vi "Send Quad Arrays to Sqlite.vi"(5 "Savepoint name":string="MySavepoint", 6 "Path to local database file *.db":path=path "C:/sqlite/sensor_data.db", 7 "TIME 1D Array REAL":dbl[](array[numeric]), 8 "error in (no error)":errorcluster, 9 "DENS 1D Array REAL":dbl[](array[numeric]), 10 "TEMP 1D Array REAL":dbl[](array[numeric]), 11 "PRESSURE 1D Array REAL":dbl[](array[numeric])) -> (0 "error out":errorcluster, 3 "Rows (Samples) Detected in input array":i32=1000)   [LabVIEW 2023]
uses:
  <vilib>/drjdpowell/SQLite Library/SQL Statement/SQL Statement.lvclass/SQL Statement.ctl
  <vilib>/drjdpowell/SQLite Library/SQL Connection/Open (path).vi
  <vilib>/drjdpowell/SQLite Library/SQL Statement/Bind Real.vi
  <vilib>/drjdpowell/SQLite Library/SQL Connection/Open (string).vi
  <vilib>/drjdpowell/SQLite Library/SQL Statement/Step.vi
  <vilib>/AdvancedString/Path To Command Line String.vi
  <vilib>/drjdpowell/SQLite Library/SQL Connection/Execute SQL (No results).vi
  <vilib>/drjdpowell/SQLite Library/SQL Statement/Error Message.vi
  <vilib>/drjdpowell/SQLite Library/SQL Connection/Connection.lvclass
  <vilib>/drjdpowell/SQLite Library/SQLite.lvlib
  <vilib>/drjdpowell/SQLite Library/Transaction Helpers/Transaction.lvlib
  <vilib>/drjdpowell/SQLite Library/SQL Statement/SQL Statement.lvclass
panel:
  in  "SQLite Command":string="CREATE TABLE IF NOT EXISTS pipe_data(\nID INTEGER PRIMARY KEY AUTOINCREMENT,\nUNIX_TIME REAL NOT NULL, \nPRESSURE REAL NOT NULL,\nTEMPERATURE REAL NOT NULL,\nDENSITY REAL NOT NULL\n);"
  # "Create a pipe_data table in sensor_data.db\nNO Indexing in this evolution.\nAdd 4 columns for data of type REAL"
  # "DATA SOURCE SELECT"
  # "THIS VI SENDS (4) 1D parameter arrays TO SQLite DATABASE TABLE pipe_data\nIt creates the table if it doesnt exist, and populates the column data with pipe parameters.\n\nAll parameter columns are forced to a NOT NULL state, any attempt at writing NULL or NaN will throw an error.\n\nNOT SURE WHAT YOU WANT TO DO ON INDEXING IN THE DB....WE CAN USE NO INDEX, INDEX ON unix_time, OR ADD A KEY FIELD. lETS DISCUSS ???????????\n\nThe first time through, the table pipe_data is created and populated with 25 samples of rando parameters.The UNIX_TIME var is not random, and should align with real times.\nThe Authority for timestamping should rest on the DAQ process to maintain accuracy, and is included in the incoming 2d array. This vi simply pushes that array time to SQLite.\nIf you run this vi again after the table has been created, the data is appended to the database in increments of 25 rows.\n\n\n\nRegarding the 14 day flush....Do you want the stale data removed from the incoming 2D array, the database, or both ?\nThroughput ?"
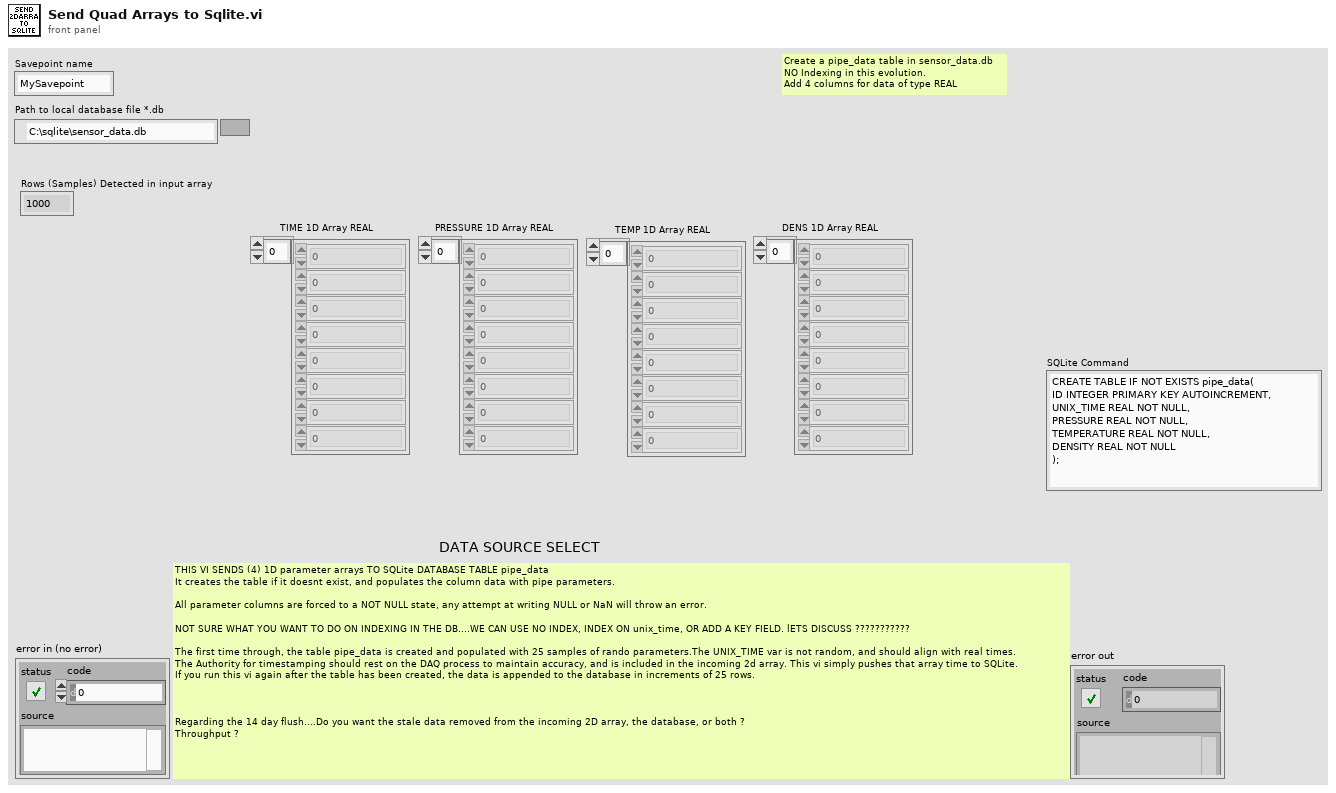
[diagram p1: front panel]
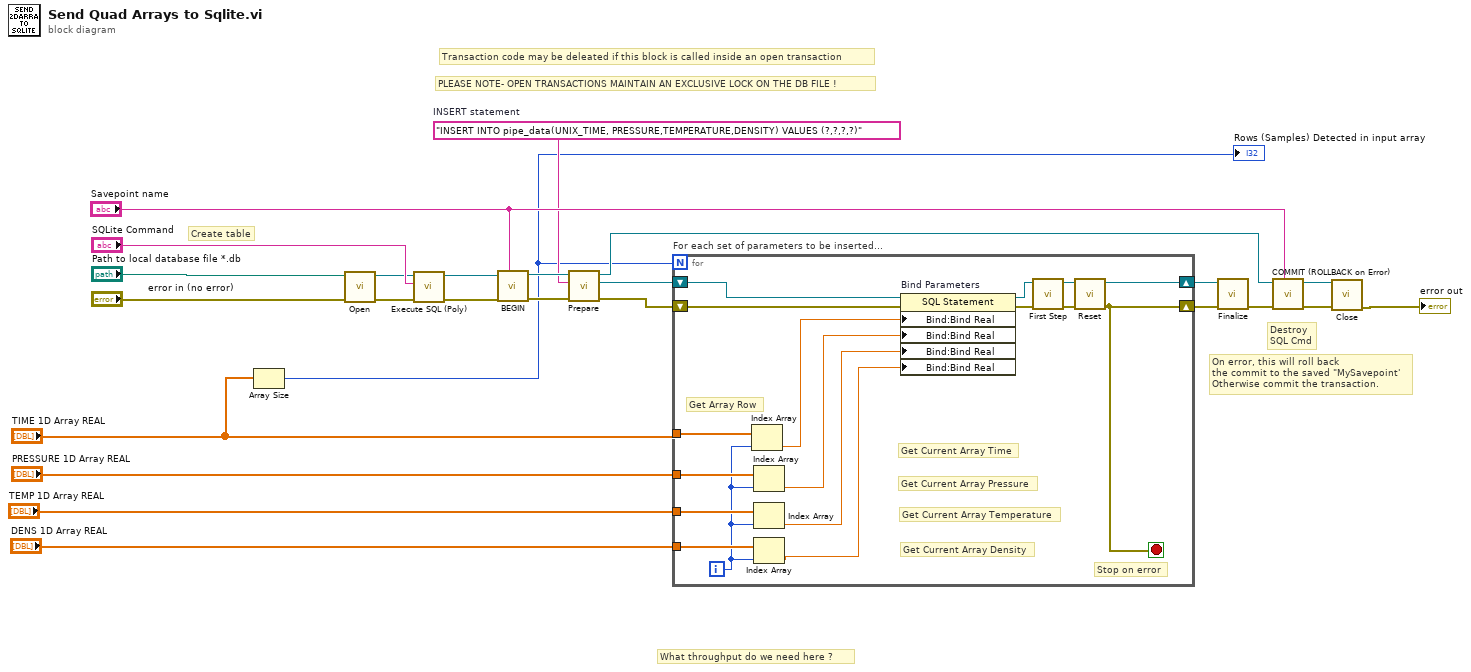
[diagram p0: block diagram]
diagram:
  w16 = "INSERT INTO pipe_data(UNIX_TIME, PRESSURE,TEMPERATURE,DENSITY) VALUES (?,?,?,?)"  # INSERT statement
  # "What throughput do we need here ?"
  # "Create table"
  # "Destroy\nSQL Cmd"
  # "On error, this will roll back\nthe commit to the saved \"MySavepoint'\nOtherwise commit the transaction."
  # "PLEASE NOTE- OPEN TRANSACTIONS MAINTAIN AN EXCLUSIVE LOCK ON THE DB FILE !"
  # "Transaction code may be deleated if this block is called inside an open transaction"
  n1 = Array Size(array="TIME 1D Array REAL") -> (size(s)=w1:i32)
  "Rows (Samples) Detected in input array" <- w1
  n2 = call-poly <vilib>:"Open.vi"("error in (no error)"="error in (no error)", "db file"="Path to local database file *.db") -> ("error out"=w24:errorcluster, "SQLite Connection"=w12:refnum<class "Connection.lvclass">)  [unwired: 8 in]
  n3 = call-poly <vilib>:"Execute SQL (Poly).vi"("error in (no error)"=w24, "SQL"="SQLite Command", "SQLite Connection in"=w12) -> ("error out"=w14:errorcluster, "SQLite Connection"=w11:refnum<class "Connection.lvclass">)  [unwired: 7 in]
  n4 = call <vilib>:"BEGIN.vi"("Savepoint name"="Savepoint name", "error in (no error)"=w14, "SQLite Connection in"=w11) -> ("error out"=w20:errorcluster, "SQLite Connection"=w19:refnum<class "Connection.lvclass">)  [unwired: 7 in]
  n5 = call <vilib>:"Prepare.vi"("error in (no error)"=w20, "SQL"=w16, "SQLite Connection in"=w19) -> ("error out"=w7:errorcluster, "SQL Statement"=w15:refnum<class "SQL Statement.lvclass">, "SQLite Connection"=w22:refnum<class "Connection.lvclass">)  [unwired: 4 in, 2 out]
  n6 = for "For each set of parameters to be inserted..." {
    N: w1 -> [_]
    shift-right: [w36] -> w17
    shift-left: w15 -> [w42]
    shift-right: [w35] -> w18
    shift-left: w7 -> [w39]
    tunnel: "TIME 1D Array REAL" -> [w31]
    tunnel: "PRESSURE 1D Array REAL" -> [w34]
    tunnel: "TEMP 1D Array REAL" -> [w33]
    tunnel: "DENS 1D Array REAL" -> [w32]
    i -> [w26]
    stop <- w35 stop-if-true
    # "Stop on error"
    # "Get Array Row"
    # "Get Current Array Density"
    # "Get Current Array Temperature"
    # "Get Current Array Pressure"
    # "Get Current Array Time"
    n7 = Index Array(array=w31, index=w26) -> (element=w30:dbl)
    n8 = Index Array(array=w34, index=w26) -> (element=w29:dbl)
    n9 = Index Array(array=w33, index=w26) -> (element=w28:dbl)
    n10 = Index Array(array=w32, index=w26) -> (element=w27:dbl)
    n11 = property on="Bind Parameters" class="SQL Statement"(reference=w42, error in=w39, "Bind:Bind Real"=w30, "Bind:Bind Real"=w29, "Bind:Bind Real"=w28, "Bind:Bind Real"=w27) -> (reference out=w41:refnum<class "SQL Statement.lvclass">, error out=w40:errorcluster)
    n12 = call <vilib>:"First Step.vi"("error in (no error)"=w40, "SQL Statement in"=w41) -> ("error out"=w38:errorcluster, "SQL Statement"=w37:refnum<class "SQL Statement.lvclass">)  [unwired: 7 in, 1 out]
    n13 = call <vilib>:"Reset.vi"("error in (no error)"=w38, "SQL Statement in"=w37) -> ("error out"=w35:errorcluster, "SQL Statement"=w36:refnum<class "SQL Statement.lvclass">)  [unwired: 8 in]
  }
  n14 = call <vilib>:"Finalize.vi"("error in (no error)"=w18, "SQL Statement in"=w17) -> ("error out"=w23:errorcluster)  [unwired: 9 in]
  n15 = call <vilib>:"COMMIT (ROLLBACK on Error).vi"("Savepoint name"="Savepoint name", "error in (no error)"=w23, "SQLite Connection in"=w22) -> ("error out"=w8:errorcluster, "SQLite Connection"=w9:refnum<class "Connection.lvclass">)  [unwired: 7 in]
  n16 = call-dynamic "Close.vi"("error in (no error)"=w8, "SQLite Connection in"=w9) -> ("error out"=→"error out":errorcluster)  [unwired: 9 in]
